vi "Clamping Position Calculations.vi"(11 "Desired Pos":T1(ring)) -> (3 "Direction":enum16{"Stop", "In", "Out"}(ring))   [LabVIEW 2014]
panel:
  out "Current Position":T1(ring)
  in  "Beam Breaker":enum16{"None", "Long", "Short"}(ring)
  in  "Min Limit":bool
  in  "Max Limit":bool
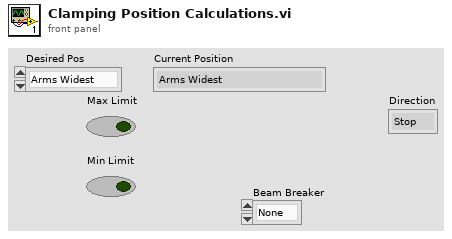
[diagram p1: front panel]
types:
  T1 = enum16{"Arms Widest", "Wide Tote", "Narrow Tote", "Arms Shortest"}
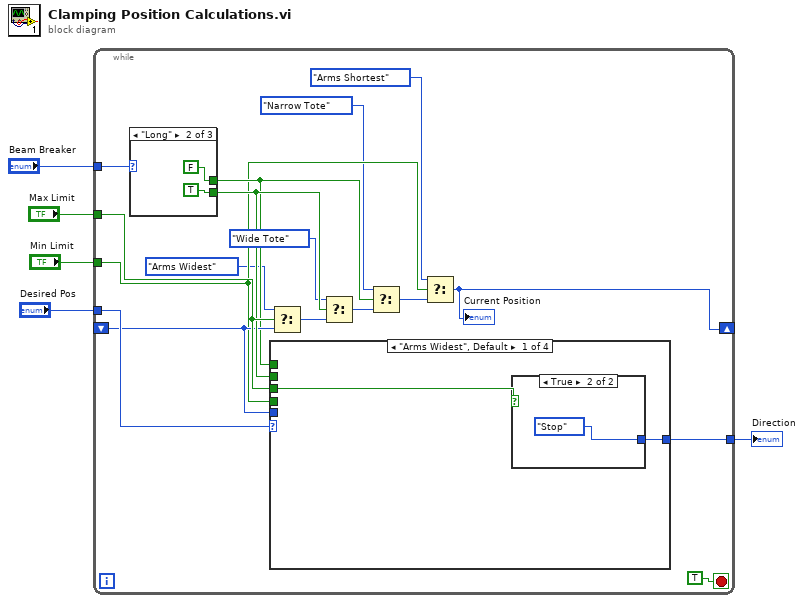
[diagram p0: block diagram]
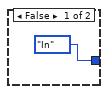
[diagram p2: hidden frame]
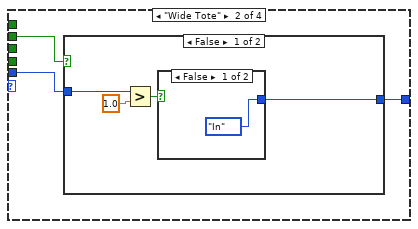
[diagram p3: hidden frame]
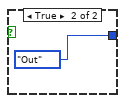
[diagram p4: hidden frame]
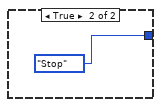
[diagram p5: hidden frame]
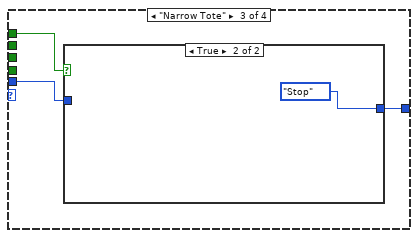
[diagram p6: hidden frame]
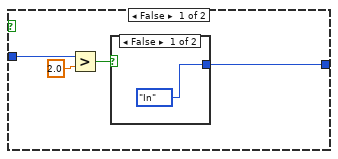
[diagram p7: hidden frame]
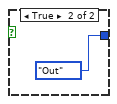
[diagram p8: hidden frame]
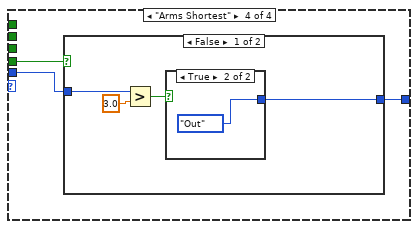
[diagram p9: hidden frame]
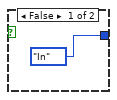
[diagram p10: hidden frame]
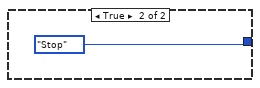
[diagram p11: hidden frame]
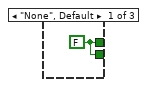
[diagram p12: hidden frame]
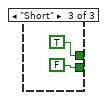
[diagram p13: hidden frame]
diagram:
  n1 = while {
    tunnel: "Max Limit" -> [w16]
    tunnel: "Min Limit" -> [w11]
    tunnel: "Beam Breaker" -> [w21]
    shift-right: [w10] -> _
    shift-left: _ -> [w13]
    tunnel: "Desired Pos" -> [w17]
    tunnel: [w15] -> w1
    stop <- TRUE stop-if-true
    n2 = case shown="\"Long\"" w21 {
      tunnel: [w57 TRUE FALSE] -> w14
      tunnel: [w57 FALSE TRUE] -> w12
      frame "None", Default {
        w57 = FALSE
      }
      frame "Long" {
      }
      frame "Short" {
      }
    }
    n3 = case shown="\"Arms Widest\", Default" w17 {
      tunnel: w16 -> [w24 _ _ _]
      tunnel: [w23 w27 w38 w48] -> w15
      tunnel: w14 -> [_ w29 _ _]
      tunnel: w13 -> [_ w28 w39 w49]
      tunnel: w12 -> [_ _ w37 _]
      tunnel: w11 -> [_ _ _ w47]
      frame "Arms Widest", Default {
        n4 = case shown="True" w24 {
          tunnel: [enum16{"Stop", "In", "Out"}."In" ("Direction 2") enum16{"Stop", "In", "Out"}."Stop" ("Direction 2")] -> w23
          frame False {
          }
          frame True {
          }
        }
      }
      frame "Wide Tote" {
        n5 = case shown="False" w29 {
          tunnel: w28 -> [w33 _]
          tunnel: [w30 enum16{"Stop", "In", "Out"}."Stop" ("Direction 2")] -> w27
          frame False {
            n6 = Greater?(x=w33, y=1.0) -> (0:w31:bool)
            n7 = case shown="False" w31 {
              tunnel: [enum16{"Stop", "In", "Out"}."In" ("Direction 2") enum16{"Stop", "In", "Out"}."Out" ("Direction 2")] -> w30
              frame False {
              }
              frame True {
              }
            }
          }
          frame True {
          }
        }
      }
      frame "Narrow Tote" {
        n8 = case shown="True" w37 {
          tunnel: w39 -> [w43 _]
          tunnel: [w41 enum16{"Stop", "In", "Out"}."Stop" ("Direction 2")] -> w38
          frame False {
            n9 = Greater?(x=w43, y=2.0) -> (0:w42:bool)
            n10 = case shown="False" w42 {
              tunnel: [enum16{"Stop", "In", "Out"}."In" ("Direction 2") enum16{"Stop", "In", "Out"}."Out" ("Direction 2")] -> w41
              frame False {
              }
              frame True {
              }
            }
          }
          frame True {
          }
        }
      }
      frame "Arms Shortest" {
        n11 = case shown="False" w47 {
          tunnel: w49 -> [w53 _]
          tunnel: [w51 enum16{"Stop", "In", "Out"}."Stop" ("Direction 2")] -> w48
          frame False {
            n12 = Greater?(x=w53, y=3.0) -> (0:w52:bool)
            n13 = case shown="True" w52 {
              tunnel: [enum16{"Stop", "In", "Out"}."In" ("Direction 2") enum16{"Stop", "In", "Out"}."Out" ("Direction 2")] -> w51
              frame False {
              }
              frame True {
              }
            }
          }
          frame True {
          }
        }
      }
    }
    n14 = Select(t=T1."Arms Widest" ("Desired Pos 2"), s=w16, f=w13) -> (s? t:f=w20:T1)
    n15 = Select(t=T1."Wide Tote" ("Desired Pos 2"), s=w14, f=w20) -> (s? t:f=w19:T1)
    n16 = Select(t=T1."Narrow Tote" ("Desired Pos 2"), s=w12, f=w19) -> (s? t:f=w18:T1)
    n17 = Select(t=T1."Arms Shortest" ("Desired Pos 2"), s=w11, f=w18) -> (s? t:f=w10:T1)
    "Current Position" <- w10
  }
  "Direction" <- w1
